vi "Path_Create_Details Word Report (SubVI).vi"(9 "שם ומק\"ט המכלל":string, 10 "מספר סידורי":string, 11 "שם הצב\"ד":string="שם הצב\"ד") -> (0 "error out":errorcluster, 2 "Path":path, 3 "NI_report out":refnum<class "NI_report.lvclass">)   [LabVIEW 2014]
uses:
  <vilib>/Utility/NIReport.llb/NI_report.lvclass
  <vilib>/addons/_office/_exclsub.llb/font.ctl
  <vilib>/Utility/NIReport.llb/Append Report Text (str wrap).vi
  <vilib>/Utility/NIReport.llb/Word/NI_Word.lvclass
  <vilib>/addons/_office/NI_ReportGenerationToolkit.lvlib
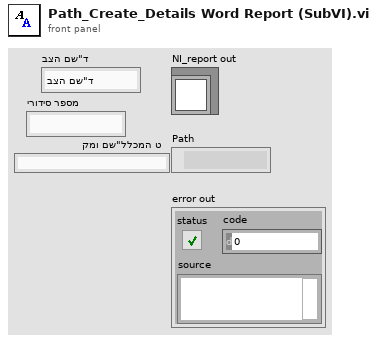
[diagram p1: front panel]
types:
  T1 = typedef "NI_ReportGenerationToolkit.lvlib/font.ctl" = cluster{"font name":string, "font size":dbl, "bold":u16, "italic":u16, "underline":u16, "strike through":u16, "font color":u32}
  T2 = enum16{"maximized", "minimized", "normal", "no change"}
  T3 = enum16{"Standard Report", "HTML", "Word", "Excel"}
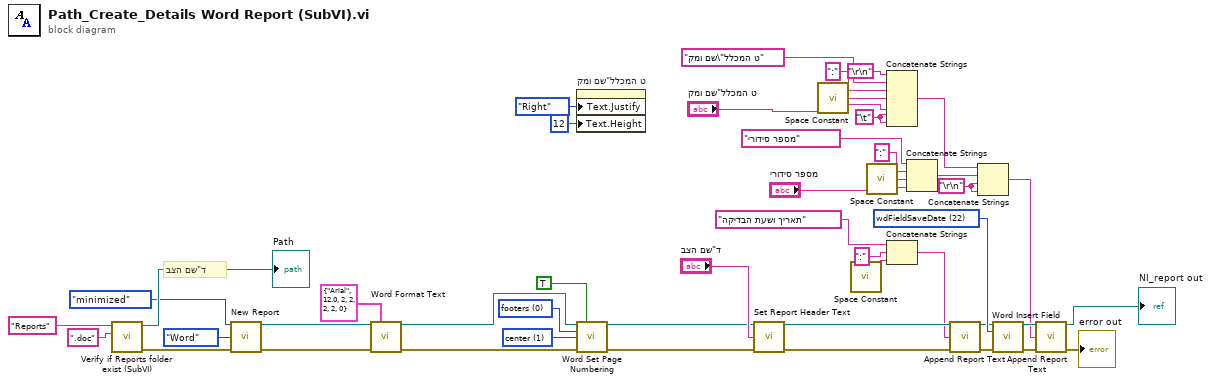
[diagram p0: block diagram]
diagram:
  w4 = "\r\n"
  w41 = "\t"
  w33 = 22 items=["wdFieldEmpty"=-1, "wdFieldRef"=3, "wdFieldIndexEntry"=4, "wdFieldFootnoteRef"=5, "wdFieldSet"=6, "wdFieldIf"=7, "wdFieldIndex"=8, "wdFieldTOCEntry"=9, "wdFieldStyleRef"=10, "wdFieldRefDoc"=11, "wdFieldSequence"=12, "wdFieldTOC"=13, "wdFieldInfo"=14, "wdFieldTitle"=15, "wdFieldSubject"=16, "wdFieldAuthor"=17, "wdFieldKeyWord"=18, "wdFieldComments"=19, "wdFieldLastSavedBy"=20, "wdFieldCreateDate"=21, "wdFieldSaveDate"=22, "wdFieldPrintDate"=23, "wdFieldRevisionNum"=24, "wdFieldEditTime"=25, "wdFieldNumPages"=26, "wdFieldNumWords"=27, "wdFieldNumChars"=28, "wdFieldFileName"=29, "wdFieldTemplate"=30, "wdFieldDate"=31, "wdFieldTime"=32, "wdFieldPage"=33, "wdFieldExpression"=34, "wdFieldQuote"=35, "wdFieldInclude"=36, "wdFieldPageRef"=37, "wdFieldAsk"=38, "wdFieldFillIn"=39, "wdFieldData"=40, "wdFieldNext"=41, "wdFieldNextIf"=42, "wdFieldSkipIf"=43, "wdFieldMergeRec"=44, "wdFieldDDE"=45, "wdFieldDDEAuto"=46, "wdFieldGlossary"=47, "wdFieldPrint"=48, "wdFieldFormula"=49, "wdFieldGoToButton"=50, "wdFieldMacroButton"=51, "wdFieldAutoNumOutline"=52, "wdFieldAutoNumLegal"=53, "wdFieldAutoNum"=54, "wdFieldImport"=55, "wdFieldLink"=56, "wdFieldSymbol"=57, "wdFieldEmbed"=58, "wdFieldMergeField"=59, "wdFieldUserName"=60, "wdFieldUserInitials"=61, "wdFieldUserAddress"=62, "wdFieldBarCode"=63, "wdFieldDocVariable"=64, "wdFieldSection"=65, "wdFieldSectionPages"=66, "wdFieldIncludePicture"=67, "wdFieldIncludeText"=68, "wdFieldFileSize"=69, "wdFieldFormTextInput"=70, "wdFieldFormCheckBox"=71, "wdFieldNoteRef"=72, "wdFieldTOA"=73, "wdFieldTOAEntry"=74, "wdFieldMergeSeq"=75, "wdFieldPrivate"=77, "wdFieldDatabase"=78, "wdFieldAutoText"=79, "wdFieldCompare"=80, "wdFieldAddin"=81, "wdFieldSubscriber"=82, "wdFieldFormDropDown"=83, "wdFieldAdvance"=84, "wdFieldDocProperty"=85, "wdFieldOCX"=87, "wdFieldHyperlink"=88, "wdFieldAutoTextList"=89, "wdFieldListNum"=90, "wdFieldHTMLActiveX"=91] ("type")
  w30 = u16 1 items=["left", "center", "right"] ("alignment (right)")
  w29 = u16 0 items=["footers", "headers"] ("position (footers)")
  # "שם הצב\"ד"
  n1 = call "Verify if Reports folder exist (SubVI).vi"("File Type"=".doc", "Folder Name"="Reports" ("string")) -> ("error out"=w45:errorcluster, "Path"=→"Path":path)  [unwired: 8 in]
  n2 = call <vilib>:"New Report.vi"("window state (normal)"=T2."minimized", "report type"=T3."Word", "error in (no error)"=w45) -> ("report out"=w35:refnum<class "NI_report.lvclass">, "error out"=w36:errorcluster)  [unwired: 11 in]
  n3 = call <vilib>:"Word Format Text.vi"("report in"=w35, "font"=T1 {"font name"="Arial", "font size"=12.0, "bold"=2, "italic"=2, "underline"=2, "strike through"=2, "font color"=0}, "error in (no error)"=w36) -> ("report out"=w26:refnum<class "NI_report.lvclass">, "error out"=w27:errorcluster)  [unwired: 11 in]
  n4 = property on="שם ומק\"ט המכלל" class="Str"("Text.Justify"=enum16{"Left", "Center", "Right"}."Right" ("Text.Justification"), "Text.Height"=u32 12 ("Text.Size:Height")) -> ()  [unwired: 2 in, 2 out]
  n5 = call <vilib>:"Word Set Page Numbering.vi"("report in"=w26, "include page x of n"=TRUE, "position (footers)"=w29, "alignment (right)"=w30, "error in (no error)"=w27) -> ("report out"=w31:refnum<class "NI_report.lvclass">, "error out"=w46:errorcluster)  [unwired: 9 in]
  n6 = call-dynamic "Set Report Header Text.vi"("report in"=w31, "center header text"="שם הצב\"ד", "error in (no error)"=w46) -> ("report out"=w19:refnum<class "NI_report.lvclass">, "error out"=w18:errorcluster)  [unwired: 11 in]
  n7 = call <vilib>:"Space Constant.vi"() -> ("String"=w12:string)
  n8 = call <vilib>:"Space Constant.vi"() -> ("String"=w7:string)
  n9 = call <vilib>:"Space Constant.vi"() -> ("String"=w11:string)
  n10 = Concatenate Strings("\r\n", "שם ומק\"ט המכלל" ("string"), ":" ("string"), w12, "שם ומק\"ט המכלל", w41, w41) -> (w5:string)
  n11 = Concatenate Strings("תאריך ושעת הבדיקה" ("string"), ":" ("string"), w7) -> (w15:string)
  n12 = Concatenate Strings("מספר סידורי" ("string"), ":" ("string"), w11, "מספר סידורי") -> (w6:string)
  n13 = call-poly <vilib>:"Append Report Text.vi"("report in"=w19, "text"=w15, "error in (no error)"=w18) -> ("report out"=w16:refnum<class "NI_report.lvclass">, "error out"=w17:errorcluster)  [unwired: 9 in, 2 out]
  n14 = Concatenate Strings(w5, w6, w4, w4) -> (w37:string)
  n15 = call <vilib>:"Word Insert Field.vi"("report in"=w16, "type"=w33, "error in (no error)"=w17) -> ("report out"=w39:refnum<class "NI_report.lvclass">, "error out"=w40:errorcluster)  [unwired: 11 in]
  n16 = call-poly <vilib>:"Append Report Text.vi"("report in"=w39, "text"=w37, "error in (no error)"=w40) -> ("report out"=→"NI_report out":refnum<class "NI_report.lvclass">, "error out"=→"error out":errorcluster)  [unwired: 9 in, 2 out]
